vi "ProcessNIData.vi"(7 "Record Data":bool, 9 "Error In":errorcluster, 10 "Queue In":refnum<queue>) -> (0 "Data Out":dbl[](array[numeric]), 1 "Error Out":errorcluster, 2 "Queue Out":refnum<queue>)   [LabVIEW 2016]
panel:
  # "ProcessNIData.vi:\n\nThis function is used to consume and process a\nNI DAQ data queue at discrete intervals. When called,\nall elements in the input queue are examined and\nformatted into a single datastream.\n\nINPUTS:\n-Record Data: boolean that controls whether to push\nprocessed data to the file output loop\n-Queue In: Queue containing all NI DAQ data since\nlast function call.\n-Error In: Error signal stream for queue operations.\n\n\nOUTPUTS:\n-Data Out: an array of floats for use by the GUI\n-Queue Out: The empty NI DAQ data queue after\noperation.\n-Error Out: Error signal stream from queue operations.\n-Output to GUI: Average values of all NI DAQ data\nfor use in the GUI."
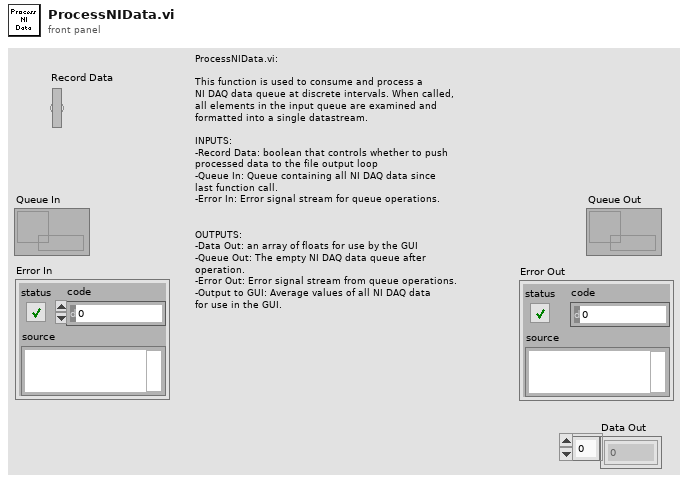
[diagram p1: front panel]
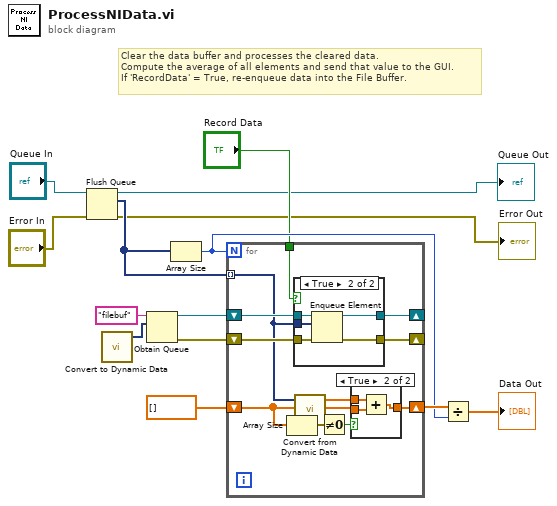
[diagram p0: block diagram]
diagram:
  # "Clear the data buffer and processes the cleared data.\nCompute the average of all elements and send that value to the GUI.\nIf 'RecordData' = True, re-enqueue data into the File Buffer."
  n1 = Flush Queue(queue="Queue In", error in (no error)="Error In") -> (queue out=→"Queue Out":refnum<queue>, remaining elements=w14:dynamicdata[], error out=→"Error Out":errorcluster)
  n2 = call "Convert to Dynamic Data"() -> ("Dynamic Data Type"=w4:dynamicdata)  [unwired: 4 in]
  n3 = Obtain Queue(name (unnamed)="filebuf", element data type=w4) -> (queue out=w2:refnum<queue>, error out=w1:errorcluster)  [unwired: 3 in, 1 out]
  n4 = Array Size(array=w14) -> (size(s)=w11:i32)
  n5 = for {
    N: w11 -> [_]
    tunnel: w14 -> [w19] mode=indexing
    shift-right: [w23] -> _
    shift-left: w2 -> [w25]
    shift-right: [w22] -> _
    shift-left: w1 -> [w24]
    shift-right: [w17] -> w12
    shift-left: dbl[] [] -> [w16]
    tunnel: "Record Data" -> [w15]
    n6 = Array Size(array=w16) -> (size(s)=w20:i32)
    n7 = case shown="True" w15 {
      tunnel: w25 -> [w27 w32]
      tunnel: w24 -> [w26 w31]
      tunnel: [w27 w30] -> w23
      tunnel: [w26 w29] -> w22
      tunnel: w19 -> [_ w28]
      frame False {
      }
      frame True {
        n8 = Enqueue Element(queue=w32, element=w28, error in (no error)=w31) -> (queue out=w30:refnum<queue>, error out=w29:errorcluster)  [unwired: 1 in, 1 out]
      }
    }
    n9 = call "Convert from Dynamic Data"("Dynamic Data Type"=w19) -> ("Array"=w18:dbl[])  [unwired: 3 in]
    n10 = Not Equal To 0?(x=w20) -> (x != 0?=w21:bool)
    n11 = case shown="True" w21 {
      tunnel: w18 -> [w33 w36]
      tunnel: w16 -> [_ w35]
      tunnel: [w33 w34] -> w17
      frame False {
      }
      frame True {
        n12 = Add(x=w36, y=w35) -> (x+y=w34:dbl[])
      }
    }
  }
  n13 = Divide(x=w12, y=w11) -> (x/y=→"Data Out":dbl[])
